vi "RANGE Parse Configuration Data.vi"(0 "all rows":string[][](array[string]), 2 "Meter Type Index":i32, 3 "Meter Size Index":i32=1, 5 "Error In":errorcluster, 7 "Heating Value Index":i32, 8 "Accuracy Reading Index":i32, 9 "Meter Present Index":i32, 11 "Accuracy Full Scale Index":i32, 13 "Set STP Register":i32) -> (10 "SLPM Error @ Zero":dbl, 12 "Heating Value (BTU/ft³)":dbl, 14 "Meter Type (Gas)":T1, 16 "Meter Size":dbl, 17 "Meter Present":bool, 18 "STP Register Set":bool, 19 "Error Out":errorcluster)   [LabVIEW 2018]
uses:
  Drivers/Omega FMA-1600A Series Gas Flow Meter/Type Definitions/FMA1600A Gas Type.ctl
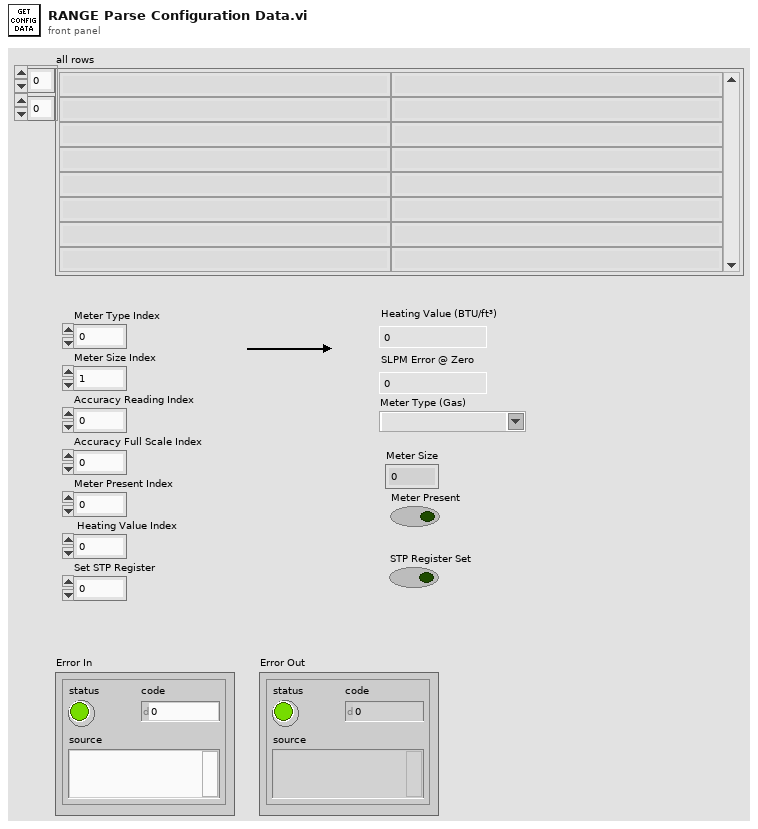
[diagram p1: front panel]
types:
  T1 = typedef "FMA1600A Gas Type.ctl" = string
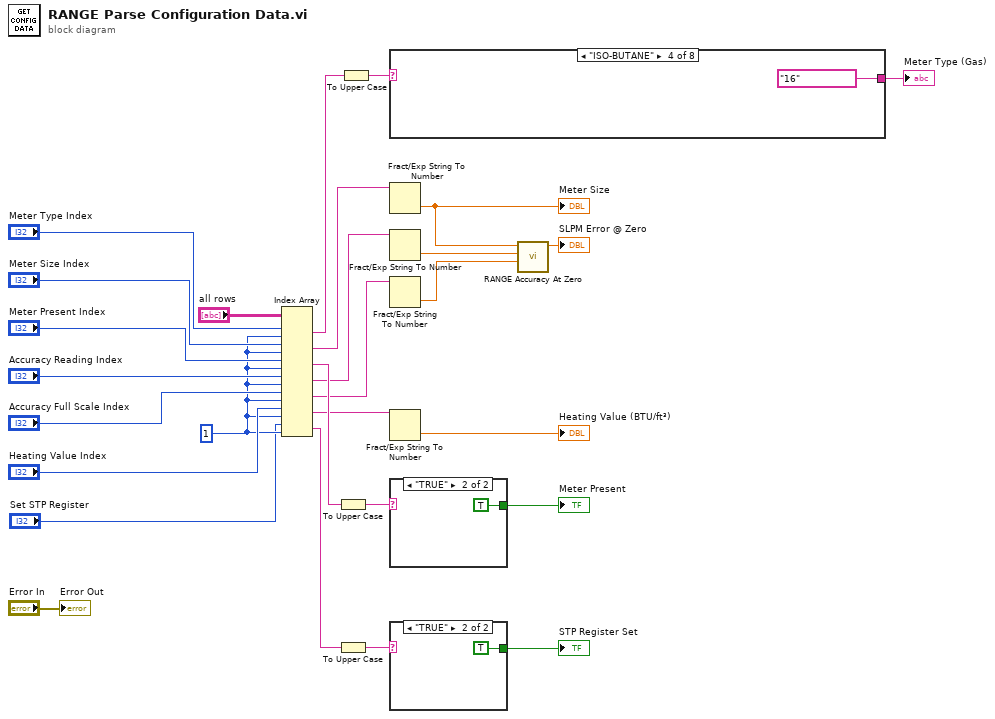
[diagram p0: block diagram]
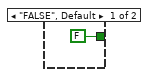
[diagram p2: hidden frame]
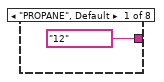
[diagram p3: hidden frame]
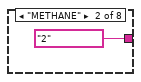
[diagram p4: hidden frame]
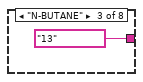
[diagram p5: hidden frame]
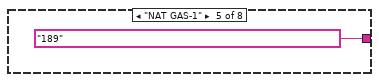
[diagram p6: hidden frame]
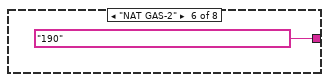
[diagram p7: hidden frame]
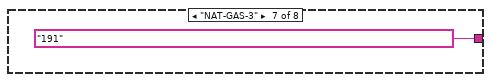
[diagram p8: hidden frame]
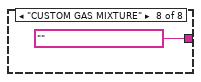
[diagram p9: hidden frame]
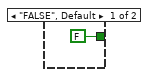
[diagram p10: hidden frame]
diagram:
  w5 = 1 ("disabled index (col)")
  n1 = Index Array(array="all rows", index (row) #1="Meter Type Index", index (col) #1=w5, index (row) #2="Meter Size Index", index (col) #2=w5, index (row) #3="Meter Present Index", index (col) #3=w5, index (row) #4="Accuracy Reading Index", index (col) #4=w5, index (row) #5="Accuracy Full Scale Index", index (col) #5=w5, index (row) #6="Heating Value Index", index (col) #6=w5, index (row) #7="Set STP Register", index (col) #7=w5) -> (element #1=w10:string, element #2=w24:string, element #3=w26:string, element #4=w17:string, element #5=w14:string, element #6=w7:string, element #7=w1:string)
  n2 = To Upper Case(1:w26) -> (0:w27:string)
  n3 = To Upper Case(1:w1) -> (0:w3:string)
  n4 = To Upper Case(1:w10) -> (0:w9:string)
  n5 = case shown="\"ISO-BUTANE\"" w9 {
    tunnel: [T1 "12" ("Meter Type (Gas)") T1 "2" ("Meter Type (Gas)") T1 "13" ("Meter Type (Gas)") T1 "16" ("Meter Type (Gas)") T1 "189" ("Meter Type (Gas)") T1 "190" ("Meter Type (Gas)") T1 "191" ("Meter Type (Gas)") T1 "" ("Meter Type (Gas)")] -> w8
    frame "PROPANE", Default {
    }
    frame "METHANE" {
    }
    frame "N-BUTANE" {
    }
    frame "ISO-BUTANE" {
    }
    frame "NAT GAS-1" {
    }
    frame "NAT GAS-2" {
    }
    frame "NAT-GAS-3" {
    }
    frame "CUSTOM GAS MIXTURE" {
    }
  }
  "Meter Type (Gas)" <- w8
  n6 = Fract/Exp String To Number(string=w24) -> (number=w15:dbl)  [unwired: 3 in, 1 out]
  "Meter Size" <- w15
  n7 = Fract/Exp String To Number(string=w17) -> (number=w16:dbl)  [unwired: 3 in, 1 out]
  n8 = Fract/Exp String To Number(string=w14) -> (number=w13:dbl)  [unwired: 3 in, 1 out]
  n9 = Fract/Exp String To Number(string=w7) -> (number=→"Heating Value (BTU/ft³)":dbl)  [unwired: 3 in, 1 out]
  n10 = case shown="\"TRUE\"" w27 {
    tunnel: [FALSE TRUE] -> w28
    frame "FALSE", Default {
    }
    frame "TRUE" {
    }
  }
  "Meter Present" <- w28
  n11 = case shown="\"TRUE\"" w3 {
    tunnel: [FALSE TRUE] -> w2
    frame "FALSE", Default {
    }
    frame "TRUE" {
    }
  }
  "STP Register Set" <- w2
  n12 = call "RANGE Accuracy At Zero.vi"("Accuracy Full Scale"=w13, "Accuracy Reading"=w16, "Meter Size"=w15) -> ("SLPMErrZero"=→"SLPM Error @ Zero":dbl)  [unwired: 8 in]
  "Error Out" <- "Error In"
